vi "Intake.vi"(8 "outakeSpeed":dbl, 9 "intakeSpeed":dbl, 10 "operatorPanel":T1, 11 "intake":T3={"DeviceStatus"={"status"=FALSE, "code"=0, "source"=""}, "Type"=enum."PWM", "PWM"={"PWM Channel"=enum."PWM 1", "DeadBand"={"Name"="", "maxPositivePwm"=0, "minPositivePwm"=0, "centerPwm"=0, "maxNegativePwm"=0, "minNegativePwm"=0, "angularRange"=0}}, "CAN"={"Device Number"=0, "SetOutput VI Ref"=variant(enum8{"Percent VBus", "Current", "Speed", "Position", "Voltage"} enum."Percent VBus"), "GetOutput VI Ref"=variant(refnum<k1> refnum), "Enable VI Ref"=variant(dbl 12.0), "Disable VI Ref"=variant(enum8{"Percent VBus", "Speed", "Position", "Slave", "Unchanged / Invalid", "Voltage Compensation", "Current", "Motion Profile"} enum."Percent VBus"), "Data"=variant}, "Invert"=FALSE, "DIO PWM"={"PWM \"Enable\" Channel"=enum."Invalid", "DIOChannel"=enum."Invalid", "PWM Rate"=0.0}}) -> (3 "intake":T3={"DeviceStatus"={"status"=FALSE, "code"=0, "source"=""}, "Type"=enum."PWM", "PWM"={"PWM Channel"=enum."PWM 1", "DeadBand"={"Name"="", "maxPositivePwm"=0, "minPositivePwm"=0, "centerPwm"=0, "maxNegativePwm"=0, "minNegativePwm"=0, "angularRange"=0}}, "CAN"={"Device Number"=0, "SetOutput VI Ref"=variant(enum8{"Percent VBus", "Current", "Speed", "Position", "Voltage"} enum."Percent VBus"), "GetOutput VI Ref"=variant(refnum<k1> refnum), "Enable VI Ref"=variant(dbl 12.0), "Disable VI Ref"=variant(enum8{"Percent VBus", "Speed", "Position", "Slave", "Unchanged / Invalid", "Voltage Compensation", "Current", "Motion Profile"} enum."Percent VBus"), "Data"=variant}, "Invert"=FALSE, "DIO PWM"={"PWM \"Enable\" Channel"=enum."Invalid", "DIOChannel"=enum."Invalid", "PWM Rate"=0.0}})   [LabVIEW 2017]
uses:
  <vilib>/Rock Robotics/WPI/MotorControl/WPI_MotorControlDeviceRef.ctl
  <vilib>/Rock Robotics/WPI/MotorControl/WPI_MotorControlType.ctl
  <vilib>/Rock Robotics/SystemInterfaces/DIO/FPGA_DIOPWMChannel.ctl
  <vilib>/Rock Robotics/WPI/PWM/WPI_PWMDeadband.ctl
  <vilib>/Rock Robotics/SystemInterfaces/DIO/FPGA_DIOChannel.ctl
  <vilib>/Rock Robotics/WPI/Joystick/WPI_JoystickDevRef.ctl
  <vilib>/Rock Robotics/WPI/Joystick/WPI_JoystickDeviceEnum.ctl
  <vilib>/Rock Robotics/WPI/ThirdParty/Phoenix-LabVIEW/Motor Controller/Controls/CTRE_Phoenix_MotorControl_ControlMode.ctl
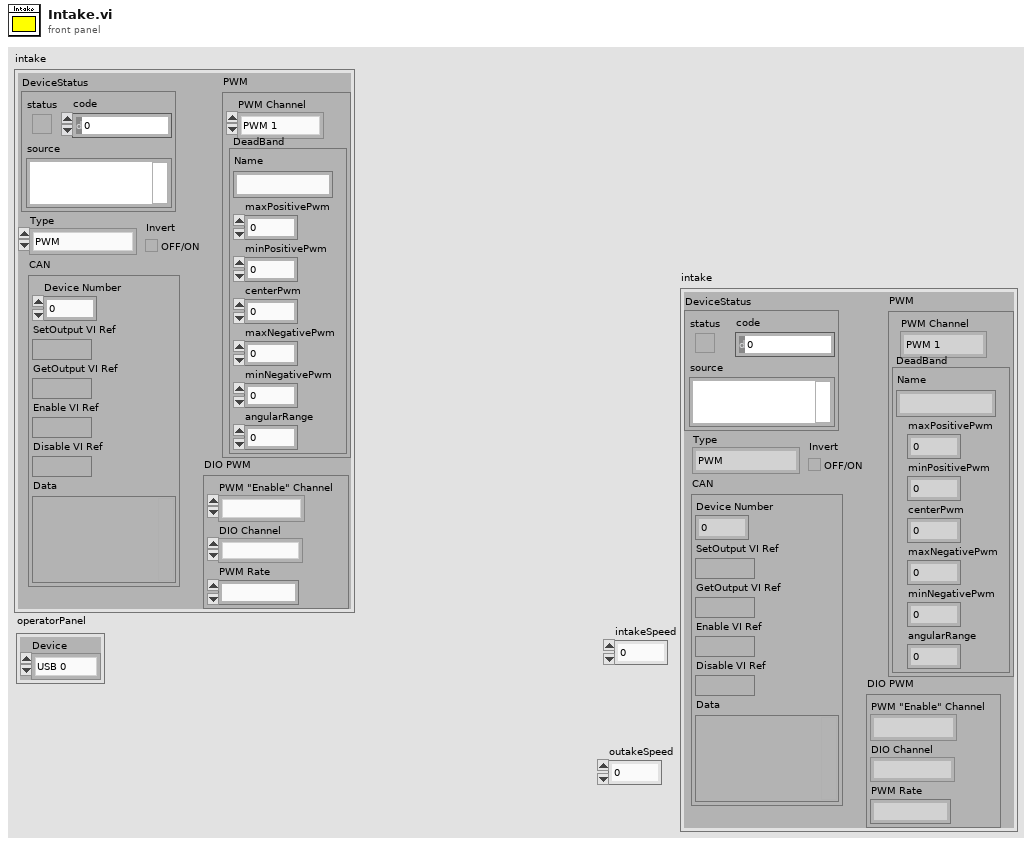
[diagram p1: front panel]
types:
  T1 = typedef "WPI_JoystickDevRef.ctl" = cluster{"Device":T2}
  T2 = typedef "WPI_JoystickDeviceEnum.ctl" = enum16{"USB 0", "USB 1", "USB 2", "USB 3", "USB 4", "USB 5"}
  T3 = typedef "WPI_MotorControlDeviceRef.ctl" = cluster{"DeviceStatus":errorcluster, "Type":T4, "PWM":cluster{"PWM Channel":T5, "DeadBand":T6}, "CAN":cluster{"Device Number":u8, "SetOutput VI Ref":variant, "GetOutput VI Ref":variant, "Enable VI Ref":variant, "Disable VI Ref":variant, "Data":variant}, "Invert":bool, "DIO PWM":cluster{"PWM \"Enable\" Channel":T5, "DIOChannel":T7, "PWM Rate":dbl}}
  T4 = typedef "WPI_MotorControlType.ctl" = enum16{"PWM", "CAN", "DIO PWM"}
  T5 = typedef "FPGA_DIOPWMChannel.ctl" = enum8{"PWM 0", "PWM 1", "PWM 2", "PWM 3", "PWM 4", "PWM 5", "PWM 6", "PWM 7", "PWM 8", "PWM 9", "PWM MXP 0", "PWM MXP 1", "PWM MXP 2", "PWM MXP 3", "PWM MXP 4", "PWM MXP 5", "PWM MXP 6", "PWM MXP 7", "PWM MXP 8", "PWM MXP 9", "Invalid"}
  T6 = typedef "WPI_PWMDeadband.ctl" = cluster{"Name":string, "maxPositivePwm":i32, "minPositivePwm":i32, "centerPwm":i32, "maxNegativePwm":i32, "minNegativePwm":i32, "angularRange":u16}
  T7 = typedef "FPGA_DIOChannel.ctl" = enum8{"DIO 0", "DIO 1", "DIO 2", "DIO 3", "DIO 4", "DIO 5", "DIO 6", "DIO 7", "DIO 8", "DIO 9", "DIO MXP 0", "DIO MXP 1", "DIO MXP 2", "DIO MXP 3", "DIO MXP 4", "DIO MXP 5", "DIO MXP 6", "DIO MXP 7", "DIO MXP 8", "DIO MXP 9", "DIO MXP 10", "DIO MXP 11", "DIO MXP 12", "DIO MXP 13", "DIO MXP 14", "DIO MXP 15", "SPI Port CS1", "SPI Port CS2", "SPI Port CS3", "SPI Port MISO", "SPI Port MOSI", "Invalid"}
  T8 = typedef "CTRE_Phoenix_MotorControl_ControlMode.ctl" = u16
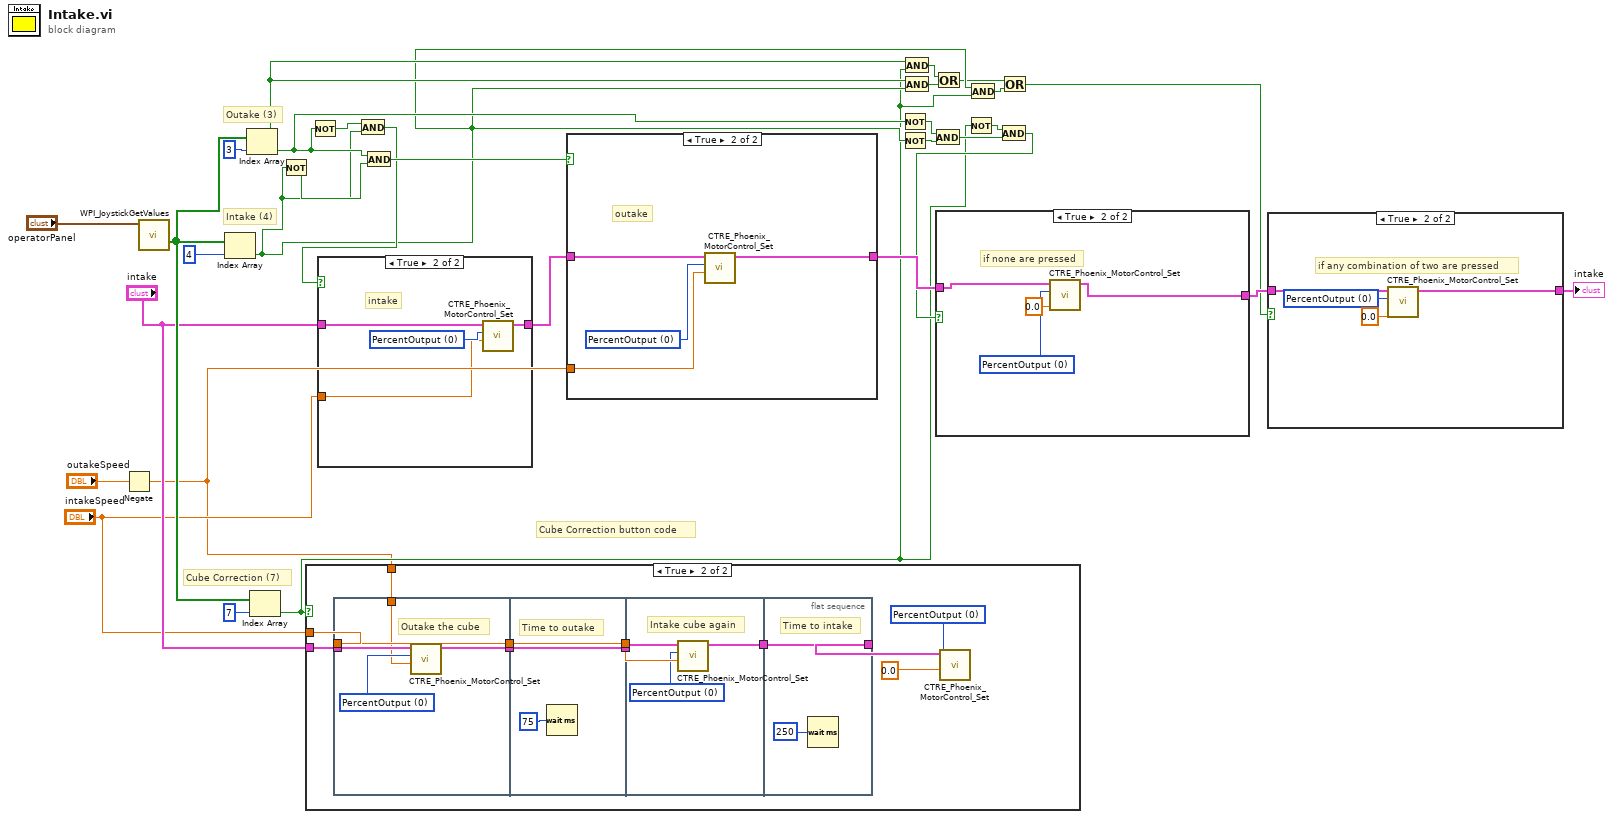
[diagram p0: block diagram]
diagram:
  # "Cube Correction button code"
  # "Cube Correction (7)"
  # "Intake (4)"
  # "Outake (3)"
  n1 = Negate(x="outakeSpeed") -> (-x=w1:dbl)
  n2 = call <vilib>:"WPI_JoystickGetValues.vi"("JoystickDevRef"="operatorPanel") -> ("Buttons"=w17:bool[])  [unwired: 6 in, 4 out]
  n3 = Index Array(array=w17, index=4) -> (element=w8:bool)
  n4 = Index Array(array=w17, index=3) -> (element=w11:bool)
  n5 = Index Array(array=w17, index=7) -> (element=w4:bool)
  n6 = Not(x=w8) -> (.not. x?=w26:bool)
  n7 = case shown="True" w4 {
    tunnel: "intake" -> [_ w41]
    tunnel: "intakeSpeed" -> [_ w36]
    tunnel: w1 -> [_ w31]
    frame False {
    }
    frame True {
      w33 = T8 0 items=["PercentOutput"=0, "Position"=1, "Velocity"=2, "Current"=3, "Follower"=5, "MotionProfile"=6, "MotionMagic"=7, "MotionMagicArc"=8, "MotionProfileArc"=10, "Disabled"=15] ("Control Mode")
      n8 = flat-sequence {
        tunnel: w41 -> [w46]
        tunnel: [w44] -> w39
        tunnel: [w43] -> w37
        tunnel: w36 -> [w43]
        tunnel: w31 -> [w42]
        tunnel: [w48] -> w40
        tunnel: w39 -> [w48]
        tunnel: [w47] -> w38
        tunnel: w37 -> [w47]
        tunnel: w40 -> [w53]
        tunnel: w38 -> [w52]
        tunnel: [w50] -> w34
        tunnel: [w54] -> w35
        tunnel: w34 -> [w54]
        frame #0 {
          w45 = T8 0 items=["PercentOutput"=0, "Position"=1, "Velocity"=2, "Current"=3, "Follower"=5, "MotionProfile"=6, "MotionMagic"=7, "MotionMagicArc"=8, "MotionProfileArc"=10, "Disabled"=15] ("Control Mode")
          # "Outake the cube"
          n9 = call <vilib>:"CTRE_Phoenix_MotorControl_Set.vi"("Output"=w42, "Control Mode"=w45, "PhoenixMotorControlDevRef"=w46) -> ("PhoenixMotorControlDevRef"=w44:T3)  [unwired: 7 in, 1 out]
        }
        frame #1 {
          # "Time to outake"
          n10 = Wait (ms)(milliseconds to wait=u32 75) -> ()  [unwired: 1 out]
        }
        frame #2 {
          w51 = T8 0 items=["PercentOutput"=0, "Position"=1, "Velocity"=2, "Current"=3, "Follower"=5, "MotionProfile"=6, "MotionMagic"=7, "MotionMagicArc"=8, "MotionProfileArc"=10, "Disabled"=15] ("Control Mode")
          # "Intake cube again"
          n11 = call <vilib>:"CTRE_Phoenix_MotorControl_Set.vi"("Output"=w52, "Control Mode"=w51, "PhoenixMotorControlDevRef"=w53) -> ("PhoenixMotorControlDevRef"=w50:T3)  [unwired: 7 in, 1 out]
        }
        frame #3 {
          # "Time to intake"
          n12 = Wait (ms)(milliseconds to wait=u32 250) -> ()  [unwired: 1 out]
        }
      }
      n13 = call <vilib>:"CTRE_Phoenix_MotorControl_Set.vi"("Output"=0.0, "Control Mode"=w33, "PhoenixMotorControlDevRef"=w35) -> ()  [unwired: 7 in, 2 out]
    }
  }
  n14 = Not(x=w11) -> (.not. x?=w21:bool)
  n15 = And(x=w21, y=w8) -> (x .and. y?=w18:bool)
  n16 = case shown="True" w18 {
    tunnel: "intakeSpeed" -> [_ w57]
    tunnel: [w56 w59] -> w28
    tunnel: "intake" -> [w56 w58]
    frame False {
    }
    frame True {
      w60 = T8 0 items=["PercentOutput"=0, "Position"=1, "Velocity"=2, "Current"=3, "Follower"=5, "MotionProfile"=6, "MotionMagic"=7, "MotionMagicArc"=8, "MotionProfileArc"=10, "Disabled"=15] ("Control Mode")
      # "intake"
      n17 = call <vilib>:"CTRE_Phoenix_MotorControl_Set.vi"("Output"=w57, "Control Mode"=w60, "PhoenixMotorControlDevRef"=w58) -> ("PhoenixMotorControlDevRef"=w59:T3)  [unwired: 7 in, 1 out]
    }
  }
  n18 = And(x=w11, y=w26) -> (x .and. y?=w22:bool)
  n19 = case shown="True" w22 {
    tunnel: w1 -> [_ w65]
    tunnel: [w61 w63] -> w25
    tunnel: w28 -> [w61 w62]
    frame False {
    }
    frame True {
      w64 = T8 0 items=["PercentOutput"=0, "Position"=1, "Velocity"=2, "Current"=3, "Follower"=5, "MotionProfile"=6, "MotionMagic"=7, "MotionMagicArc"=8, "MotionProfileArc"=10, "Disabled"=15] ("Control Mode")
      # "outake"
      n20 = call <vilib>:"CTRE_Phoenix_MotorControl_Set.vi"("Output"=w65, "Control Mode"=w64, "PhoenixMotorControlDevRef"=w62) -> ("PhoenixMotorControlDevRef"=w63:T3)  [unwired: 7 in, 1 out]
    }
  }
  n21 = Not(x=w11) -> (.not. x?=w24:bool)
  n22 = Not(x=w8) -> (.not. x?=w23:bool)
  n23 = And(x=w11, y=w4) -> (x .and. y?=w10:bool)
  n24 = And(x=w11, y=w8) -> (x .and. y?=w9:bool)
  n25 = And(x=w24, y=w23) -> (x .and. y?=w14:bool)
  n26 = Or(x=w10, y=w9) -> (x .or. y?=w7:bool)
  n27 = Not(x=w4) -> (.not. x?=w13:bool)
  n28 = And(x=w8, y=w4) -> (x .and. y?=w6:bool)
  n29 = And(x=w13, y=w14) -> (x .and. y?=w12:bool)
  n30 = case shown="True" w12 {
    tunnel: w25 -> [w66 w70]
    tunnel: [w66 w67] -> w20
    frame False {
    }
    frame True {
      w69 = T8 0 items=["PercentOutput"=0, "Position"=1, "Velocity"=2, "Current"=3, "Follower"=5, "MotionProfile"=6, "MotionMagic"=7, "MotionMagicArc"=8, "MotionProfileArc"=10, "Disabled"=15] ("Control Mode")
      # "if none are pressed"
      n31 = call <vilib>:"CTRE_Phoenix_MotorControl_Set.vi"("Output"=0.0, "Control Mode"=w69, "PhoenixMotorControlDevRef"=w70) -> ("PhoenixMotorControlDevRef"=w67:T3)  [unwired: 7 in, 1 out]
    }
  }
  n32 = Or(x=w7, y=w6) -> (x .or. y?=w5:bool)
  n33 = case shown="True" w5 {
    tunnel: w20 -> [w71 w75]
    tunnel: [w71 w74] -> w19
    frame False {
    }
    frame True {
      w73 = T8 0 items=["PercentOutput"=0, "Position"=1, "Velocity"=2, "Current"=3, "Follower"=5, "MotionProfile"=6, "MotionMagic"=7, "MotionMagicArc"=8, "MotionProfileArc"=10, "Disabled"=15] ("Control Mode")
      # "if any combination of two are pressed"
      n34 = call <vilib>:"CTRE_Phoenix_MotorControl_Set.vi"("Output"=0.0, "Control Mode"=w73, "PhoenixMotorControlDevRef"=w75) -> ("PhoenixMotorControlDevRef"=w74:T3)  [unwired: 7 in, 1 out]
    }
  }
  "intake" <- w19
